vi "VI Server_TREE_ItemSymbol_SET.vi"(4 "Symbol":i32=1, 6 "Active Cell:Active Column Number":i32=3, 7 "Label":string, 8 "error in":errorcluster, 9 "Tree.Ref":refnum<vi>, 10 "SingleInstance":bool=TRUE, 11 "VI Server.RefsCluster":T1) -> (0 "error out":errorcluster, 1 "Tree.Ref.DUP":refnum<vi>, 3 "VI Server.RefsCluster.DUP":T1)   [LabVIEW 2020]
uses:
  VI Server_TypeDefs/VI Server_RefsCluster.ctl
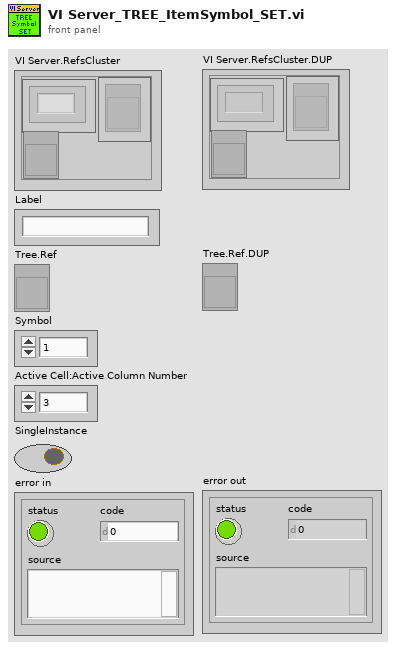
[diagram p1: front panel]
types:
  T1 = typedef "VI Server_RefsCluster.ctl" = cluster{"Labels":string[], "Refs":refnum<vi>[], "VI Ref":refnum<vi>}
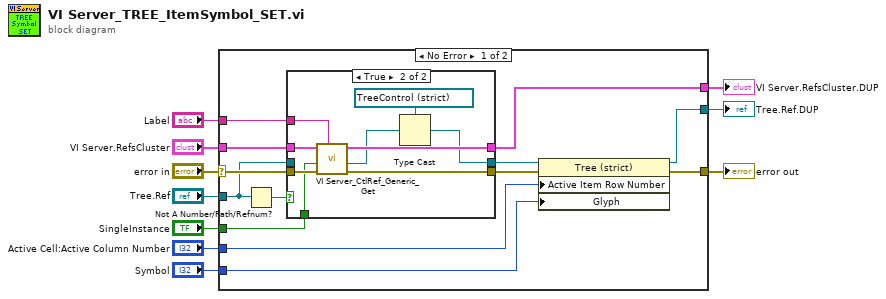
[diagram p0: block diagram]
diagram:
  n1 = case shown="No Error" "error in" {
    selector: "error in" -> [w23 w37]
    tunnel: [w14 w37] -> w9
    tunnel: "VI Server.RefsCluster" -> [w22 w36]
    tunnel: [w21 w36] -> w7
    tunnel: "Label" -> [w20 _]
    tunnel: "SingleInstance" -> [w19 _]
    tunnel: [w13 _] -> w4
    tunnel: "Tree.Ref" -> [w17 _]
    tunnel: "Active Cell:Active Column Number" -> [w12 _]
    tunnel: "Symbol" -> [w11 _]
    frame No Error {
      n2 = Not A Number/Path/Refnum?(number/path/refnum=w17) -> (NaN/Path/Refnum?=w18:bool)
      n3 = case shown="True" w18 {
        tunnel: w23 -> [w26 w35]
        tunnel: w22 -> [w24 w34]
        tunnel: [w24 w33] -> w21
        tunnel: w20 -> [_ w32]
        tunnel: w19 -> [_ w30]
        tunnel: [w25 w28] -> w16
        tunnel: [w26 w27] -> w15
        tunnel: w17 -> [w25 _]
        frame False {
        }
        frame True {
          n4 = call "VI Server_CtlRef_Generic_Get.vi"("Control.Label"=w32, "error in"=w35, "SingleInstance"=w30, "VI Server.RefsCluster"=w34) -> ("error out"=w27:errorcluster, "Control.Ref.Generic"=w31:refnum<vi>, "VI Server.RefsCluster.DUP"=w33:T1)  [unwired: 5 in]
          n5 = Type Cast(type=refnum<vi> refnum ("Tree"), x=w31) -> (*(type *) &x=w28:refnum<vi>)
        }
      }
      n6 = property on="Property Node" class="Tree (strict)"(reference=w16, error in=w15, "Active Item Row Number"=w12, "Glyph"=w11) -> (reference out=w13:refnum<vi>, error out=w14:errorcluster)
    }
    frame Error {
    }
  }
  "VI Server.RefsCluster.DUP" <- w7
  "error out" <- w9
  "Tree.Ref.DUP" <- w4
